vi "Stack_sequence.vi"() -> ()   [LabVIEW 2017]
doc: "This VI is used to determine the string to output to the weather station based on the current temperature and limit settings.\n\nInputs: Current Temperature (DBL), Minimum Temperature (DBL), and Maximum Temperature (DBL).\nOutputs: Warning Text (string) and Warning? (Boolean)."
panel:
  out "Error Out":errorcluster
  in  "Error In":errorcluster
  out "Warning Text":string="No Warning"
  out "Warning?":bool
  in  "Min Temperature":dbl
  in  "Max Temperature":dbl
  in  "Current Temperature":dbl
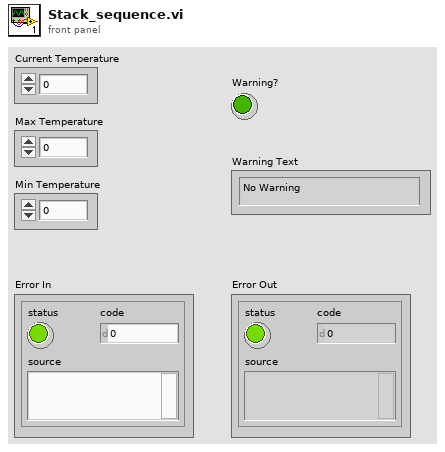
[diagram p1: front panel]
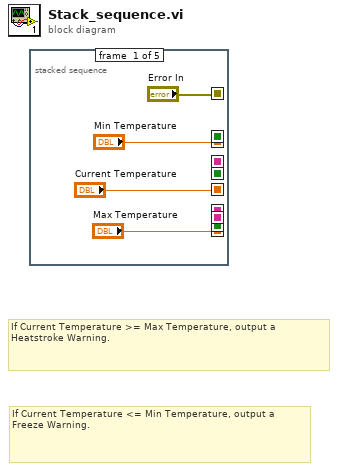
[diagram p0: block diagram]
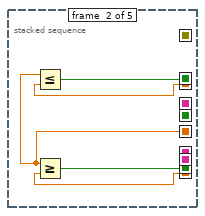
[diagram p2: hidden frame]
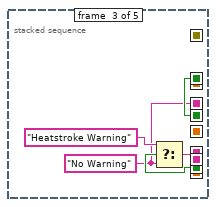
[diagram p3: hidden frame]
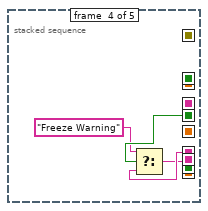
[diagram p4: hidden frame]
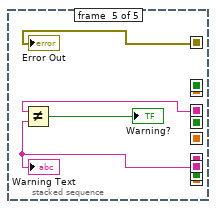
[diagram p5: hidden frame]
diagram:
  # "If Current Temperature >= Max Temperature, output a Heatstroke Warning."
  # "If Current Temperature <= Min Temperature, output a Freeze Warning."
  n1 = stacked-sequence {
    seq-local: ["Min Temperature" _ _ _ _] -> [_ w10 _ _ _]
    seq-local: ["Current Temperature" _ _ _ _] -> [_ w8 _ _ _]
    seq-local: ["Max Temperature" _ _ _ _] -> [_ w9 _ _ _]
    seq-local: ["Error In" _ _ _ _] -> [_ w5 _ _ _]
    seq-local: [_ w7 _ _ _] -> [_ _ w16 _ _]
    seq-local: [_ w6 _ _ _] -> [_ _ w13 _ _]
    seq-local: [_ w5 _ _ _] -> [_ _ w12 _ _]
    seq-local: [_ _ w14 _ _] -> [_ _ _ w22 _]
    seq-local: [_ _ w13 _ _] -> [_ _ _ w21 _]
    seq-local: [_ _ w12 _ _] -> [_ _ _ w19 _]
    seq-local: [_ _ w11 _ _] -> [_ _ _ w17 _]
    seq-local: [_ _ _ w20 _] -> [_ _ _ _ w25]
    seq-local: [_ _ _ w19 _] -> [_ _ _ _ w24]
    seq-local: [_ _ _ w17 _] -> [_ _ _ _ w23]
    frame #0 {
    }
    frame #1 {
      n2 = Less Or Equal?(x=w8, y=w10) -> (x <= y?=w6:bool)
      n3 = Greater Or Equal?(x=w8, y=w9) -> (x >= y?=w7:bool)
    }
    frame #2 {
      w11 = "No Warning" ("f")
      n4 = Select(t="Heatstroke Warning", s=w16, f=w11) -> (s? t:f=w14:string)
    }
    frame #3 {
      n5 = Select(t="Freeze Warning", s=w21, f=w22) -> (s? t:f=w20:string)
    }
    frame #4 {
      n6 = Not Equal?(x=w23, y=w25) -> (x != y?=→"Warning?":bool)
      "Warning Text" <- w25
      "Error Out" <- w24
    }
  }
